vi "OpenFITSHead.vi"(0 "file path":path=path "D:/freigabe/test256x300.fits", 1 "error in":errorcluster) -> (2 "FITS file":T2={"fits refnum"=refnum, "Byte-Reihenfolge (0:Big-Endian, 2:LSB)"=enum."native, host order"}, 3 "FITS":T1={"BITPIX"=8, "NAXIS"=2, "NAXIS1"=100, "NAXIS2"=100, "NAXIS3"=100, "BZERO"=0.0, "BSCALE"=1.0}, 5 "error out":errorcluster)   [LabVIEW 2011]
panel:
  out "Array":string[](array[string])=["SIMPLE  =                    T / Created by ImageJ FITS_Writer                  ", "BITPIX  =                   16 / number of bits per data pixel                  ", "NAXIS   =                    2 / number of data axes                            ", "NAXIS1  =                 256  / length of data axis 1                          ", "NAXIS2  =                 300  / length of data axis 2                          ", "BZERO   =                32768 / data range offset                              ", "BSCALE  =                    1 / default scaling factor                         ", "END                                                                             ", "                                                                                ", "                                                                                ", "                                                                                ", "                                                                                ", "                                                                                ", "                                                                                ", "                                                                                ", "                                                                                ", "                                                                                ", "                                                                                ", "                                                                                ", "                                                                                ", "                                                                                ", "                                                                                ", "                                                                                ", "                                                                                ", "                                                                                ", "                                                                                ", "                                                                                ", "                                                                                ", "                                                                                ", "                                                                                ", "                                                                                ", "                                                                                ", "                                                                                ", "                                                                                ", "                                                                                ", "                                                                                "]
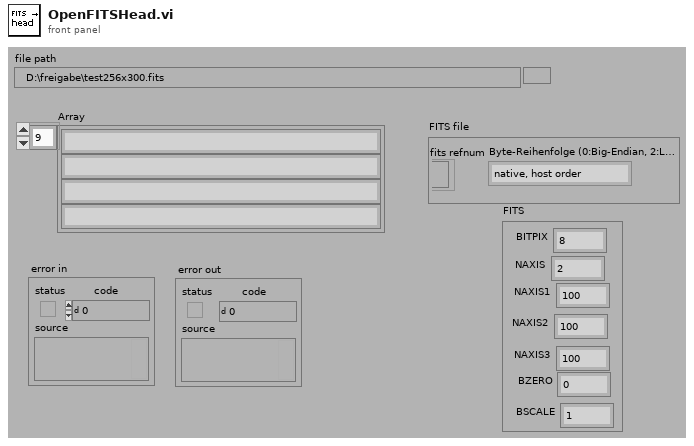
[diagram p1: front panel]
types:
  T1 = cluster{"BITPIX":i16, "NAXIS":i16, "NAXIS1":u16, "NAXIS2":u16, "NAXIS3":u16, "BZERO":dbl, "BSCALE":dbl}
  T2 = cluster{"fits refnum":refnum<file>, "Byte-Reihenfolge (0:Big-Endian, 2:LSB)":enum16{"big-endian, network order", "native, host order", "little-endian"}}
  T3 = enum16{"big-endian, network order", "native, host order", "little-endian"}
  T4 = enum16{"read/write", "read-only", "write-only", "write-only (truncate)"}
  T5 = cluster{"[0]":i32, "[1]":i32, "[2]":i32, "[3]":i32, "[4]":i32, "[5]":i32, "[6]":i32}
  T6 = cluster{"refnum out":refnum<file>, "Byte-Reihenfolge (0:Big-Endian, Netzwerkreihenfolge)":enum16{"big-endian, network order", "native, host order", "little-endian"}}
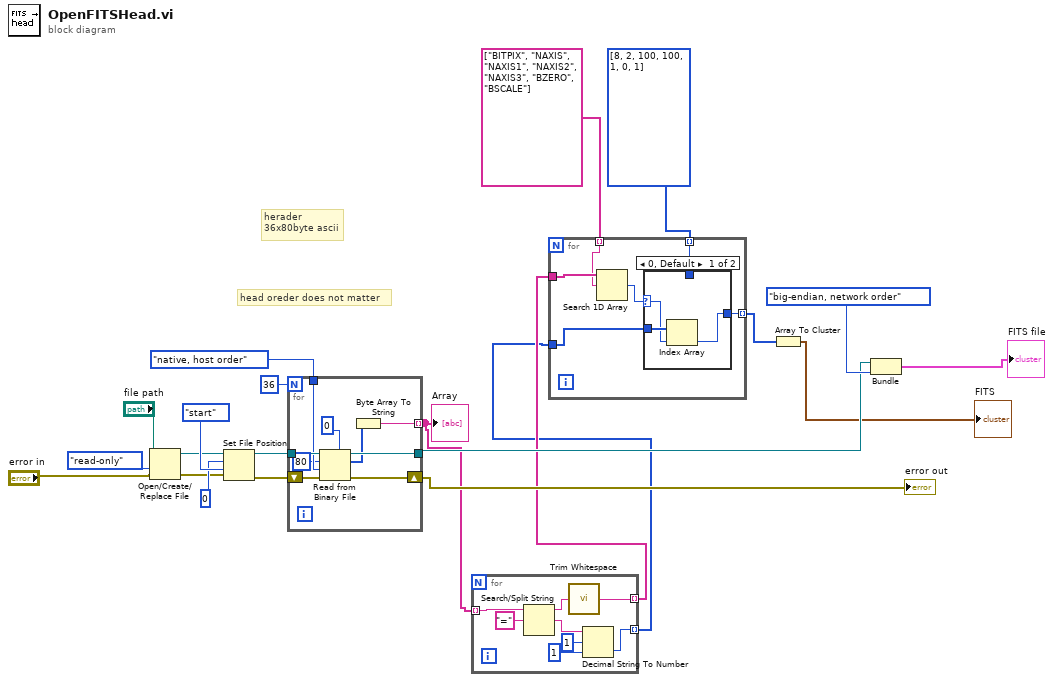
[diagram p0: block diagram]
diagram:
  # "head oreder does not matter"
  # "herader\n36x80byte ascii"
  n1 = Open/Create/Replace File(file path (use dialog)="file path", error in="error in", access (0:read/write)=T4."read-only" ("open mode (0)")) -> (refnum out=w17:refnum<file>, error out=w16:errorcluster)  [unwired: 4 out]
  n2 = Set File Position(offset (in bytes) (0)=0 ("IFDoffset"), refnum=w17, from (0:start)=enum16{"start", "end", "current"}."start" ("pos mode (0:2)"), error in=w16) -> (refnum out=w14:refnum<file>, error out=w13:errorcluster)
  n3 = for {
    N: 36 -> [_]
    tunnel: w14 -> [w30]
    tunnel: T3."native, host order" ("Byte-Reihenfolge (0:Big-Endian, Netzwerkreihenfolge)") -> [w28]
    shift-right: [w26] -> w10
    shift-left: w13 -> [w29]
    tunnel: [w25] -> w9
    tunnel: [w23] -> w7 mode=indexing
    n4 = Read from Binary File(5:u8 0 ("byte stream type"), 8:w29, 9:w28, 10:80 ("count (1)"), 11:w30) -> (0:w26:errorcluster, 2:w24:u8[], 3:w25:refnum<file>)  [unwired: 2 out]
    n5 = Byte Array To String(unsigned byte array=w24) -> (string=w23:string)
  }
  "error out" <- w10
  "Array" <- w7
  n6 = for {
    tunnel: w7 -> [w39] mode=indexing
    tunnel: [w34] -> w5 mode=indexing
    tunnel: [w33] -> w6 mode=indexing
    n7 = Search/Split String(string=w39, search string/char (-)="=") -> (substring before match=w37:string, match + rest of string=w36:string)  [unwired: 1 in, 1 out]
    n8 = call <vilib>:"Trim Whitespace.vi"("string"=w37) -> ("trimmed string"=w33:string)  [unwired: 1 in]
    n9 = Decimal String To Number(string=w36, offset=1, default (0L)=1 ("default (0 I32)")) -> (number=w34:i32)  [unwired: 1 out]
  }
  n10 = for {
    tunnel: w6 -> [w45]
    tunnel: w5 -> [w40]
    tunnel: string[] ["BITPIX", "NAXIS", "NAXIS1", "NAXIS2", "NAXIS3", "BZERO", "BSCALE"] -> [w44] mode=indexing
    tunnel: i32[] [8, 2, 100, 100, 1, 0, 1] -> [w42] mode=indexing
    tunnel: [w41] -> w2 mode=indexing
    n11 = Search 1D Array(1D array=w45, element=w44) -> (index of element=w43:i32)  [unwired: 1 in]
    n12 = case shown="0, Default" w43 {
      selector: w43 -> [w47 _]
      tunnel: w42 -> [_ w49]
      tunnel: [w46 w49] -> w41
      tunnel: w40 -> [w48 _]
      frame 0, Default {
        n13 = Index Array(array=w48, index=w47) -> (element=w46:i32)
      }
      frame -1 {
      }
    }
  }
  n14 = Array To Cluster(array=w2) -> (cluster=→"FITS":T5)
  n15 = Bundle("refnum out"=w9, "Byte-Reihenfolge (0:Big-Endian, Netzwerkreihenfolge)"=T3."big-endian, network order") -> (→"FITS file":T6)  [unwired: 1 out]
